vi "Synapse Initialize.vi"(8 "error in (no error)":errorcluster, 9 "timeout (60 s)":dbl[unit]=60.0, 10 "Unique id":string="CCD1") -> (0 "error out":errorcluster, 1 "activeYPixels":i32=256, 2 "activeXPixels":i32=1024, 3 "JYCCDLib.IJYCCDReqd":refnum<k7>, 4 "Name":string="ccd de test", 5 "Firmware Version":string="V1.89  CCD_3000", 7 "Disable shutter?":bool)   [LabVIEW 2017]
doc: "Initializes the CCD (if not already initialized), including setting the default time units to milliseconds and reading out the active X and Y areas of the CCD in pixels. Also returns the name and firmware version of the instrument."
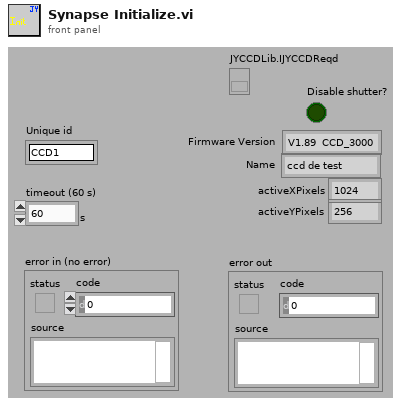
[diagram p1: front panel]
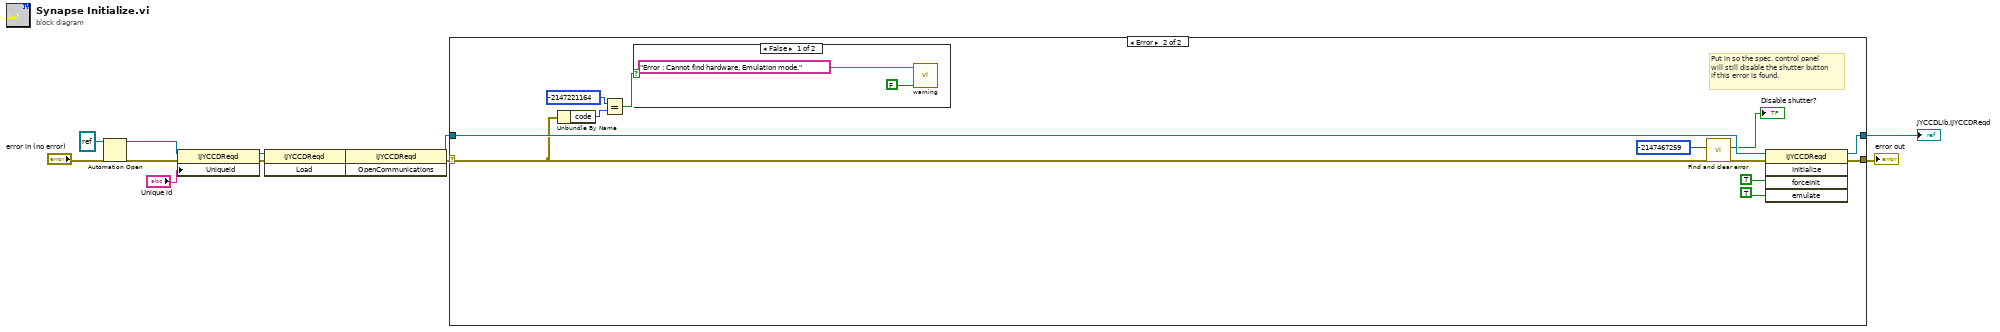
[diagram p0: block diagram]
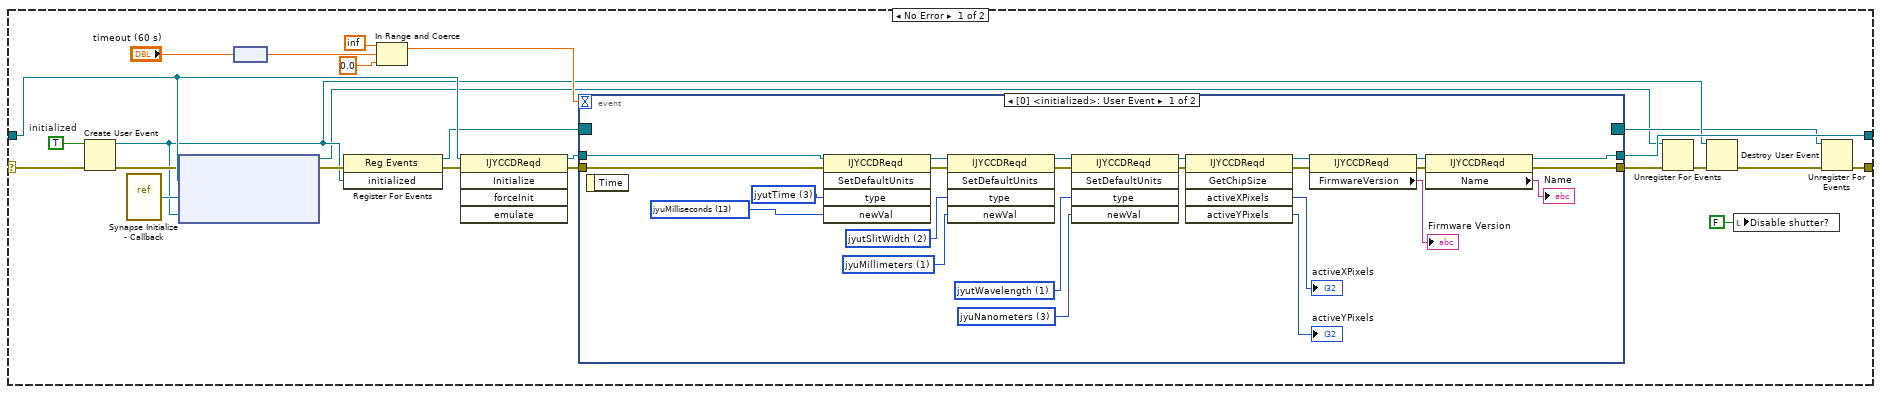
[diagram p2: hidden frame]
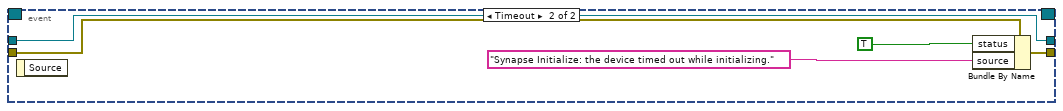
[diagram p3: hidden frame]
diagram:
  n1 = Automation Open(error in (no error)="error in (no error)", Automation Refnum=refnum<k7> refnum ("JYCCDLib.IJYCCDReqd")) -> (Automation Refnum=w4:refnum<k7>, error out=w3:errorcluster)  [unwired: 2 out]
  n2 = property class="IJYCCDReqd"(reference=w4, error in=w3, "Uniqueid"="Unique id") -> (reference out=w8:refnum<k7>, error out=w7:errorcluster)
  n3 = invoke class="IJYCCDReqd" method="Load"(reference=w8, error in=w7) -> (reference out=w10:refnum<k7>, error out=w13:errorcluster)  [unwired: 1 in, 1 out]
  n4 = invoke class="IJYCCDReqd" method="OpenCommunications"(reference=w10, error in=w13) -> (reference out=w12:refnum<k7>, error out=w11:errorcluster)  [unwired: 1 in, 1 out]
  n5 = case shown="Error" w11 {
    selector: w11 -> [w24 w71]
    tunnel: [w35 w77] -> w5
    tunnel: [w18 w76] -> w2
    tunnel: w12 -> [w27 w78]
    frame No Error {
      w28 = TRUE  # initialized
      n6 = Create User Event(user event datatype=w28, error in=w24) -> (user event=w20:refnum<user-event>, error out=w23:errorcluster)
      n7 = vi-ref "Synapse Initialize - Callback.vi"() -> ("vi reference"=w29:refnum<vi>)
      n8 = node(w23, w27, w29, w20) -> (w17:refnum<k27>, w26:errorcluster)  [unwired: 1 in]
      n9 = node("timeout (60 s)") -> (w31:dbl)
      n10 = register-events(error in=w26, w20) -> (reference out=w22:refnum<event-registration>, error out=w25:errorcluster)  [unwired: 1 in]
      n11 = In Range and Coerce(upper limit=inf, x=w31, lower limit=0.0) -> (coerced(x)=w30:dbl)  [unwired: 1 out]
      n12 = invoke class="IJYCCDReqd" method="Initialize"(reference=w27, error in=w25) -> (reference out=w37:refnum<k7>, error out=w36:errorcluster)  [unwired: 3 in, 3 out]
      n13 = event shown="[0] <initialized>: User Event" {
        selector: w22 -> [_ _]
        dyn-events: [_ _] -> w19
        timeout: w30 -> [_ _]
        tunnel: w37 -> [w49 w66]
        tunnel: w36 -> [w48 w65]
        tunnel: [w55 w66] -> w35
        tunnel: [w54 w62] -> w16
        event User Event {
          w44 = 3 items=["jyuUndefined", "jyuMillimeters", "jyuMicrons", "jyuNanometers", "jyuAngstroms", "jyuPicometers", "jyuBandpass", "jyuSteps", "jyuWavenumbers", "jyuDeltaWavenumbers", "jyuElectronVolts", "jyuNanoseconds", "jyuMicroseconds", "jyuMilliseconds", "jyuSeconds", "jyuMinutes", "jyuHours", "jyuVolts", "jyuMillivolts", "jyuMicrovolts", "jyuAmperes", "jyuMilliAmps", "jyuMicroAmps", "jyuCounts", "jyuCountsPerSecond", "jyuDegreesCelcius", "jyuDegreesFahrenheit", "jyuDegreesKelvin", "jyuPixels", "jyuTotalUnitsPlusOne"] ("newVal")
          w45 = 1 items=["jyuUndefined", "jyuMillimeters", "jyuMicrons", "jyuNanometers", "jyuAngstroms", "jyuPicometers", "jyuBandpass", "jyuSteps", "jyuWavenumbers", "jyuDeltaWavenumbers", "jyuElectronVolts", "jyuNanoseconds", "jyuMicroseconds", "jyuMilliseconds", "jyuSeconds", "jyuMinutes", "jyuHours", "jyuVolts", "jyuMillivolts", "jyuMicrovolts", "jyuAmperes", "jyuMilliAmps", "jyuMicroAmps", "jyuCounts", "jyuCountsPerSecond", "jyuDegreesCelcius", "jyuDegreesFahrenheit", "jyuDegreesKelvin", "jyuPixels", "jyuTotalUnitsPlusOne"] ("newVal")
          w46 = 1 items=["jyutUndefined", "jyutWavelength", "jyutSlitWidth", "jyutTime", "jyutTemperature", "jyutDataUnits", "jyutSpatial", "jyutTotalTypesPlusOne"] ("type")
          w47 = 2 items=["jyutUndefined", "jyutWavelength", "jyutSlitWidth", "jyutTime", "jyutTemperature", "jyutDataUnits", "jyutSpatial", "jyutTotalTypesPlusOne"] ("type")
          w50 = 13 items=["jyuUndefined", "jyuMillimeters", "jyuMicrons", "jyuNanometers", "jyuAngstroms", "jyuPicometers", "jyuBandpass", "jyuSteps", "jyuWavenumbers", "jyuDeltaWavenumbers", "jyuElectronVolts", "jyuNanoseconds", "jyuMicroseconds", "jyuMilliseconds", "jyuSeconds", "jyuMinutes", "jyuHours", "jyuVolts", "jyuMillivolts", "jyuMicrovolts", "jyuAmperes", "jyuMilliAmps", "jyuMicroAmps", "jyuCounts", "jyuCountsPerSecond", "jyuDegreesCelcius", "jyuDegreesFahrenheit", "jyuDegreesKelvin", "jyuPixels", "jyuTotalUnitsPlusOne"] ("newVal")
          w51 = 3 items=["jyutUndefined", "jyutWavelength", "jyutSlitWidth", "jyutTime", "jyutTemperature", "jyutDataUnits", "jyutSpatial", "jyutTotalTypesPlusOne"] ("type")
          n14 = event-data() -> ()  [unwired: 2 out]
          n15 = invoke class="IJYCCDReqd" method="SetDefaultUnits"(reference=w49, error in=w48, "type"=w51, "newVal"=w50) -> (reference out=w43:refnum<k7>, error out=w42:errorcluster)  [unwired: 1 in, 3 out]
          n16 = invoke class="IJYCCDReqd" method="SetDefaultUnits"(reference=w43, error in=w42, "type"=w47, "newVal"=w45) -> (reference out=w41:refnum<k7>, error out=w40:errorcluster)  [unwired: 1 in, 3 out]
          n17 = invoke class="IJYCCDReqd" method="SetDefaultUnits"(reference=w41, error in=w40, "type"=w46, "newVal"=w44) -> (reference out=w39:refnum<k7>, error out=w38:errorcluster)  [unwired: 1 in, 3 out]
          n18 = invoke class="IJYCCDReqd" method="GetChipSize"(reference=w39, error in=w38) -> (reference out=w53:refnum<k7>, error out=w52:errorcluster, "activeXPixels"=→"activeXPixels":i32, "activeYPixels"=→"activeYPixels":i32)  [unwired: 3 in, 1 out]
          n19 = property class="IJYCCDReqd"(reference=w53, error in=w52) -> (reference out=w59:refnum<k7>, error out=w60:errorcluster, "FirmwareVersion"=→"Firmware Version":string)
          n20 = property class="IJYCCDReqd"(reference=w59, error in=w60) -> (reference out=w55:refnum<k7>, error out=w54:errorcluster, "Name"=→"Name":string)
        }
        event Timeout {
          n21 = event-data() -> ()  [unwired: 2 out]
          n22 = Bundle By Name(cluster=w65, "status"=TRUE, "source"="Synapse Initialize: the device timed out while initializing.") -> (w62:errorcluster)
        }
      }
      n23 = Unregister For Events(event registration refnum=w17, error in=w16) -> (error out=w15:errorcluster)
      n24 = Destroy User Event(user event=w20, error in=w15) -> (error out=w21:errorcluster)
      n25 = local write "Disable shutter?"(FALSE ("Disable shutter?")) -> ()
      n26 = Unregister For Events(event registration refnum=w19, error in=w21) -> (error out=w18:errorcluster)
    }
    frame Error {
      # "Put in so the spec. control panel will still disable the shutter button if this error is found."
      n27 = Unbundle By Name(w71) -> ("code"=w70:i32)
      n28 = Equal?(x=-2147221164, y=w70) -> (x = y?=w68:bool)
      n29 = case shown="False" w68 {
        frame False {
          n30 = call "warning.vi"("with cancel ?"=FALSE, "Text"="Error : Cannot find hardware, Emulation mode." ("message")) -> ()  [unwired: 2 in, 1 out]
        }
        frame True {
        }
      }
      n31 = call "Find and clear error.vi"("error in (no error)"=w71, "error code"=-2147467259) -> ("error out"=w72:errorcluster, "error found?"=→"Disable shutter?":bool)  [unwired: 8 out]
      n32 = invoke class="IJYCCDReqd" method="Initialize"(reference=w78, error in=w72, "forceInit"=TRUE, "emulate"=TRUE) -> (reference out=w77:refnum<k7>, error out=w76:errorcluster)  [unwired: 1 in, 3 out]
    }
  }
  "JYCCDLib.IJYCCDReqd" <- w5
  "error out" <- w2
